vi "Find_Full_Equal_Points_and_Correct-2.vi"(4 "error IN":errorcluster, 7 "[IN] Clusters for Re\nconstructed Tracks":T1) -> (0 "error OUT":errorcluster, 3 "[OUT] Clusters for Re\nconstructed Tracks":T1)   [LabVIEW 2013]
doc: "The subVI corrects observed problem with reconstructing of resolved tracks: time-to-time, in severe conditions (big max displacement, many objects), the problem with copying of resolved subtracks"
panel:
  out "# of Track":i32
  out "Index in Track":i32
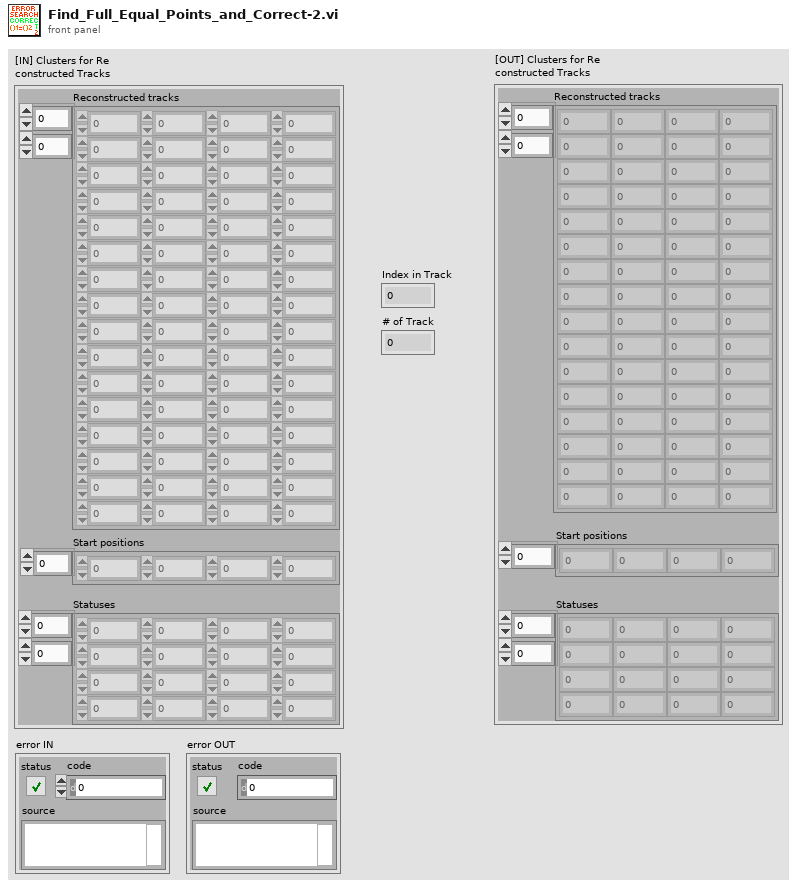
[diagram p1: front panel]
types:
  T1 = cluster{"Reconstructed tracks":dbl[][], "Start positions":i32[], "Statuses":i16[][]}
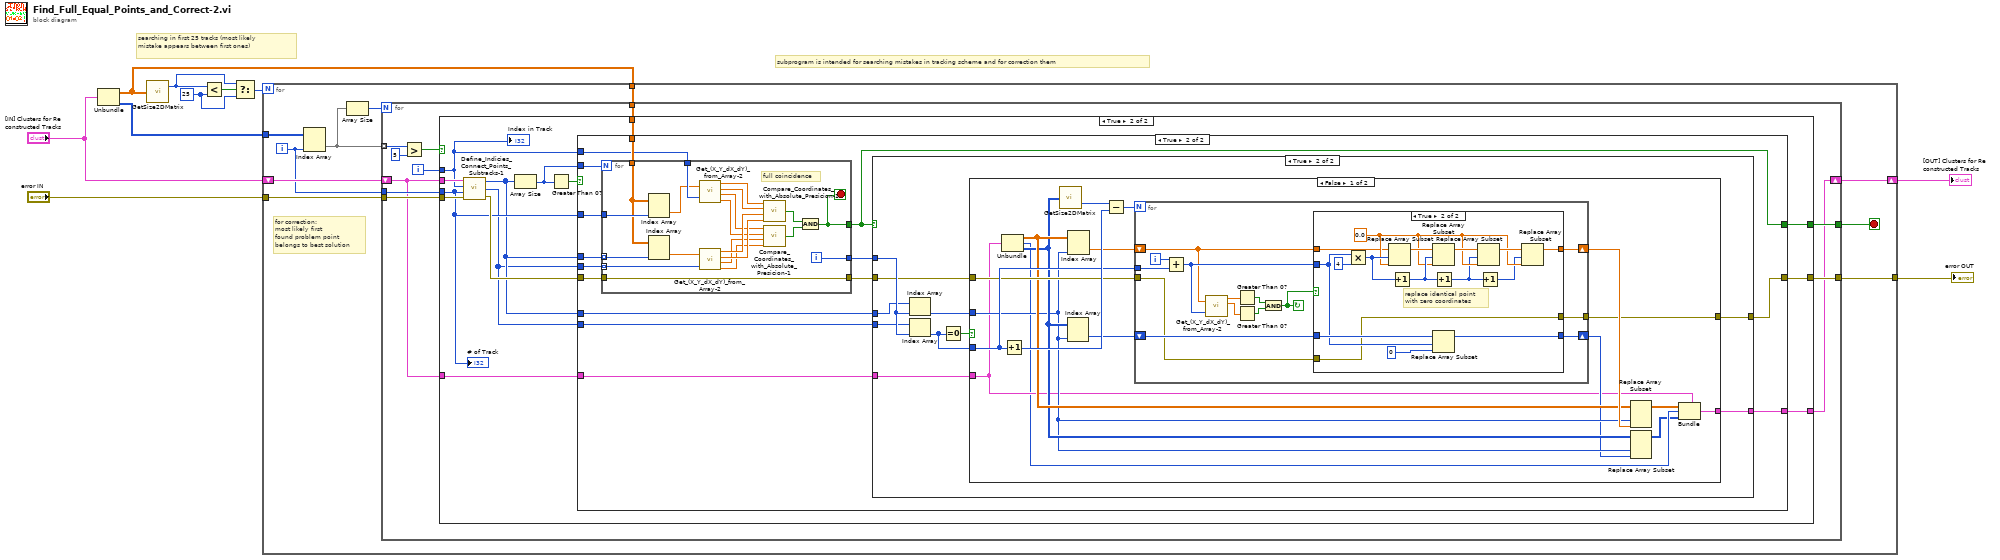
[diagram p0: block diagram]
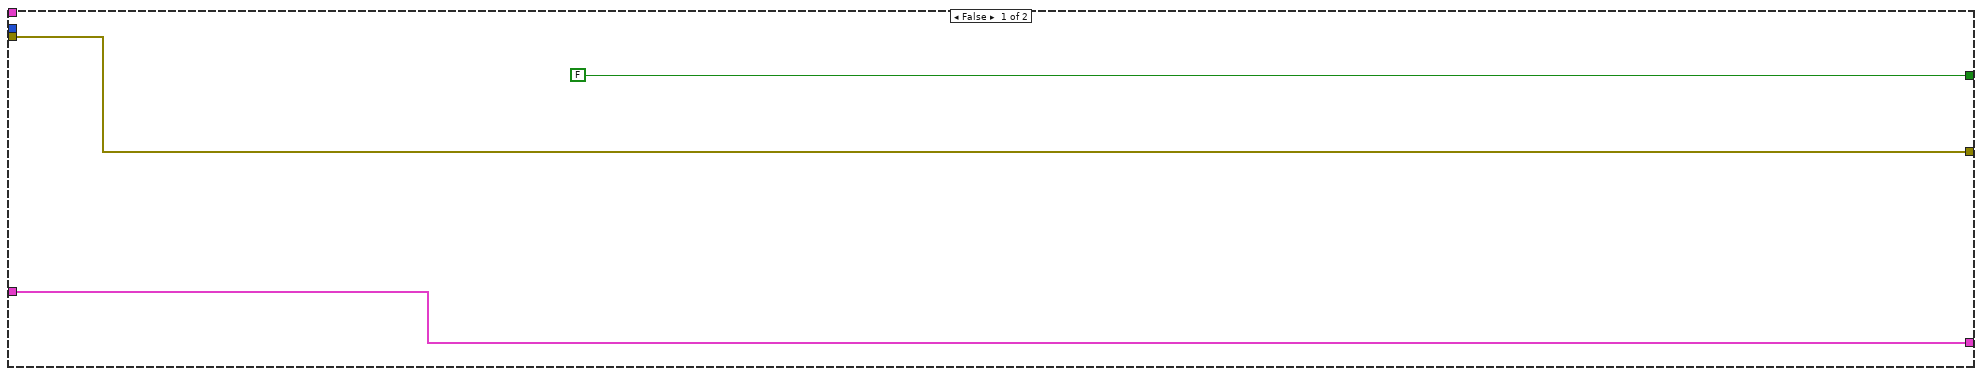
[diagram p2: hidden frame]
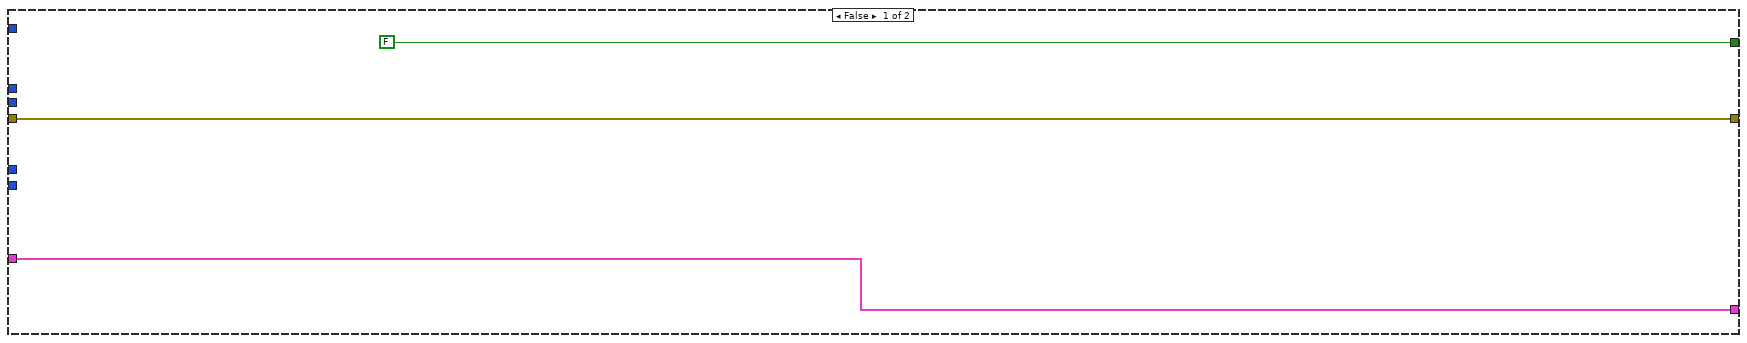
[diagram p3: hidden frame]
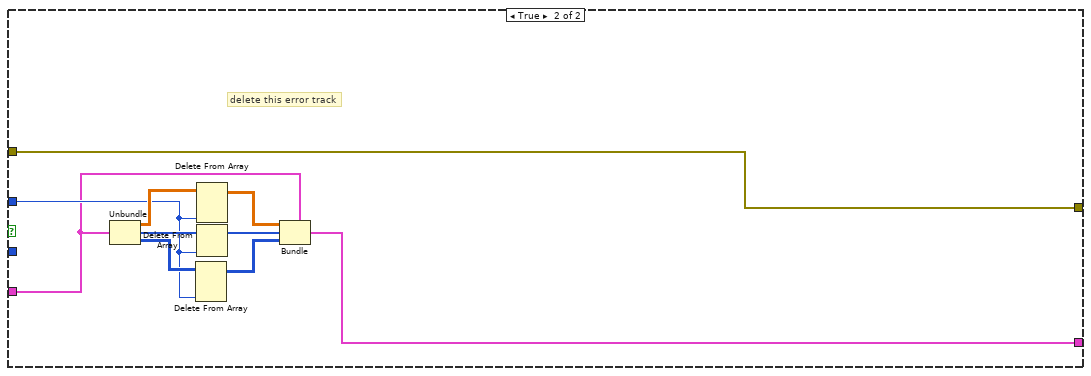
[diagram p6: hidden frame]
diagram:
  w4 = 25 ("y")
  # "searching in first 25 tracks (most likely \nmistake appears between first ones)"
  # "subprogram is intended for searching mistakes in tracking scheme and for correction them"
  n1 = Unbundle("[IN] Clusters for Re\nconstructed Tracks") -> ("Reconstructed tracks"=w1:dbl[][], "Statuses"=w2:i16[][])  [unwired: 1 out]
  n2 = call "GetSize2DMatrix.vi"("Array IN (2D)"=w1) -> ("# Cols"=w5:i32)  [unwired: 1 out]
  n3 = Less?(x=w5, y=w4) -> (x < y?=w6:bool)
  n4 = Select(t=w5, s=w6, f=w4) -> (s? t:f=w3:i32)
  n5 = for {
    N: w3 -> [_]
    tunnel: w2 -> [w20]
    tunnel: "error IN" -> [w16]
    tunnel: w1 -> [w14]
    tunnel: [w12] -> w8
    shift-right: [w11] -> w7
    shift-left: "[IN] Clusters for Re\nconstructed Tracks" -> [w17]
    i -> [w15]
    stop <- w13 stop-if-true
    # "for correction:\nmost likely first\nfound problem point\nbelongs to best solution"
    n6 = Index Array(array=w20, index (col)=w15) -> (element=w18:i16[])  [unwired: 1 in]
    n7 = Array Size(array=w18) -> (size(s)=w19:i32)
    n8 = for {
      N: w19 -> [_]
      tunnel: w18 -> [w28] mode=indexing
      tunnel: w16 -> [w29]
      tunnel: w15 -> [w26]
      tunnel: w14 -> [w25]
      tunnel: [w24] -> w13
      tunnel: [w23] -> w12
      shift-right: [w21] -> w11
      shift-left: w17 -> [w22]
      i -> [w27]
      n9 = Greater?(x=w28, y=i16 5) -> (0:w30:bool)
      n10 = case shown="True" w30 {
        tunnel: w22 -> [_ w48]
        tunnel: w29 -> [w33 w47]
        tunnel: w27 -> [_ w41]
        tunnel: w26 -> [_ w42]
        tunnel: w25 -> [_ w43]
        tunnel: [FALSE w40] -> w24
        tunnel: [w33 w39] -> w23
        tunnel: w22 -> [w32 w38]
        tunnel: [w32 w35] -> w21
        frame False {
        }
        frame True {
          n11 = call "Define_Indicies_Connect_Points_Subtracks-1.vi"("error IN"=w47, "[IN] Index of track with\n(problem displacement)"=w42, "[IN] Index of problem\ndisplacement inside track"=w41, "[IN] Track group"=w48) -> ("error OUT"=w44:errorcluster, "[OUT] Index of \nconnected dots\ninside the track"=w36:i32[], "[OUT] Index of connected\ntracks with problem dot"=w37:i32[])
          n12 = Array Size(array=w37) -> (size(s)=w46:i32)
          n13 = Greater Than 0?(x=w46) -> (x > 0?=w45:bool)
          n14 = case shown="True" w45 {
            tunnel: w46 -> [_ w66]
            tunnel: w37 -> [_ w65]
            tunnel: w36 -> [_ w64]
            tunnel: w44 -> [w50 w63]
            tunnel: w43 -> [_ w62]
            tunnel: w42 -> [_ w61]
            tunnel: w41 -> [_ w60]
            tunnel: [FALSE w54] -> w40
            tunnel: [w50 w53] -> w39
            tunnel: w38 -> [w49 w59]
            tunnel: w37 -> [_ w56]
            tunnel: w36 -> [_ w55]
            tunnel: [w49 w52] -> w35
            frame False {
            }
            frame True {
              n15 = for {
                N: w66 -> [_]
                tunnel: w65 -> [w155] mode=indexing
                tunnel: w64 -> [w153] mode=indexing
                tunnel: w63 -> [w142]
                tunnel: w62 -> [w156]
                tunnel: w61 -> [w159]
                tunnel: w60 -> [w158]
                tunnel: [w141] -> w54
                tunnel: [w142] -> w57
                tunnel: [w140] -> w58
                i -> [w140]
                stop <- w141 stop-if-true
                # "full coincidence"
                n16 = Index Array(array=w156, index (col)=w159) -> (element=w157:dbl[])  [unwired: 1 in]
                n17 = Index Array(array=w156, index (col)=w155) -> (element=w154:dbl[])  [unwired: 1 in]
                n18 = call "Get_(X_Y_dX_dY)_from_Array-2.vi"("(X,Y,dX,dY)"=w157, "Index of Displacement"=w158) -> ("X"=w152:dbl, "Y"=w151:dbl, "dX"=w148:dbl, "dY"=w147:dbl)
                n19 = call "Get_(X_Y_dX_dY)_from_Array-2.vi"("(X,Y,dX,dY)"=w154, "Index of Displacement"=w153) -> ("X"=w150:dbl, "Y"=w149:dbl, "dX"=w146:dbl, "dY"=w145:dbl)
                n20 = call "Compare_Coordinates_with_Absolute_Presicion-1.vi"("X 1"=w152, "Y 1"=w151, "X 2"=w150, "Y 2"=w149) -> ("[OUT] Same coordinates?"=w144:bool)  [unwired: 1 in]
                n21 = call "Compare_Coordinates_with_Absolute_Presicion-1.vi"("X 1"=w148, "Y 1"=w147, "X 2"=w146, "Y 2"=w145) -> ("[OUT] Same coordinates?"=w143:bool)  [unwired: 1 in]
                n22 = And(x=w144, y=w143) -> (x .and. y?=w141:bool)
              }
              n23 = case shown="True" w54 {
                tunnel: w59 -> [w68 w78]
                tunnel: w58 -> [_ w77]
                tunnel: w57 -> [w67 w76]
                tunnel: w56 -> [_ w75]
                tunnel: w55 -> [_ w74]
                tunnel: [w68 w70] -> w52
                tunnel: [w67 w69] -> w53
                frame False {
                }
                frame True {
                  n24 = Index Array(array=w75, index=w77) -> (element=w72:i32)
                  n25 = Index Array(array=w74, index=w77) -> (element=w71:i32)
                  n26 = Equal To 0?(x=w71) -> (x = 0?=w73:bool)
                  n27 = case shown="False" w73 {
                    tunnel: w76 -> [w90 w130]
                    tunnel: w78 -> [w84 w135]
                    tunnel: w72 -> [w86 w136]
                    tunnel: [w80 w131] -> w70
                    tunnel: w71 -> [w92 _]
                    tunnel: [w79 w130] -> w69
                    frame False {
                      n28 = Unbundle(w84) -> ("Reconstructed tracks"=w88:dbl[][], "Start positions"=w82:i32[], "Statuses"=w87:i16[][])
                      n29 = Increment(x=w92) -> (x+1=w95:i32)
                      n30 = call "GetSize2DMatrix.vi"("Array IN (2D)"=w87) -> ("# Rows"=w96:i32)  [unwired: 1 out]
                      n31 = Index Array(array=w87, index (col)=w86) -> (element=w91:i16[])  [unwired: 1 in]
                      n32 = Index Array(array=w88, index (col)=w86) -> (element=w93:dbl[])  [unwired: 1 in]
                      n33 = Subtract(x=w96, y=w95) -> (x-y=w94:i32)
                      n34 = for {
                        N: w94 -> [_]
                        shift-right: [w108] -> w89
                        shift-left: w93 -> [w104]
                        tunnel: w92 -> [w109]
                        shift-right: [w99] -> w85
                        shift-left: w91 -> [w100]
                        tunnel: w90 -> [w98]
                        tunnel: [w97] -> w79
                        i -> [w110]
                        stop <- w101 continue-if-true
                        n35 = Add(x=w110, y=w109) -> (x+y=w107:i32)
                        n36 = call "Get_(X_Y_dX_dY)_from_Array-2.vi"("(X,Y,dX,dY)"=w104, "Index of Displacement"=w107) -> ("X"=w106:dbl, "Y"=w105:dbl)  [unwired: 2 out]
                        n37 = Greater Than 0?(x=w106) -> (x > 0?=w103:bool)
                        n38 = Greater Than 0?(x=w105) -> (x > 0?=w102:bool)
                        n39 = And(x=w103, y=w102) -> (x .and. y?=w101:bool)
                        n40 = case shown="True" w101 {
                          tunnel: [w113 w120] -> w108
                          tunnel: w107 -> [_ w117]
                          tunnel: w104 -> [w113 w119]
                          tunnel: w100 -> [w112 w118]
                          tunnel: [w112 w115] -> w99
                          tunnel: w98 -> [w111 w114]
                          tunnel: [w111 w114] -> w97
                          frame False {
                          }
                          frame True {
                            w123 = 0.0 ("new element/subarray")
                            # "replace identical point \nwith zero coordinates"
                            n41 = Multiply(x=w117, y=4) -> (x*y=w127:i32)
                            n42 = Replace Array Subset(array=w119, new element=w123, index=w127) -> (w128:dbl[])
                            n43 = Increment(x=w127) -> (x+1=w125:i32)
                            n44 = Replace Array Subset(array=w128, new element=w123, index=w125) -> (w126:dbl[])
                            n45 = Replace Array Subset(array=w118, new element=i16 0 ("new element/subarray"), index=w117) -> (w115:i16[])
                            n46 = Increment(x=w125) -> (x+1=w122:i32)
                            n47 = Replace Array Subset(array=w126, new element=w123, index=w122) -> (w124:dbl[])
                            n48 = Increment(x=w122) -> (x+1=w121:i32)
                            n49 = Replace Array Subset(array=w124, new element=w123, index=w121) -> (w120:dbl[])
                          }
                        }
                      }
                      n50 = Replace Array Subset(array=w88, new element=w89, index (col)=w86) -> (w83:dbl[][])  [unwired: 1 in]
                      n51 = Replace Array Subset(array=w87, new element=w85, index (col)=w86) -> (w81:i16[][])  [unwired: 1 in]
                      n52 = Bundle(cluster=w84, "Reconstructed tracks"=w83, "Start positions"=w82, "Statuses"=w81) -> (w80:T1)
                    }
                    frame True {
                      # "delete this error track"
                      n53 = Unbundle(w135) -> ("Reconstructed tracks"=w139:dbl[][], "Start positions"=w138:i32[], "Statuses"=w137:i16[][])
                      n54 = Delete From Array(array=w137, index (col)=w136) -> (array with subset deleted=w132:i16[][])  [unwired: 2 in, 1 out]
                      n55 = Delete From Array(array=w139, index (col)=w136) -> (array with subset deleted=w134:dbl[][])  [unwired: 2 in, 1 out]
                      n56 = Delete From Array(array=w138, index=w136) -> (array with subset deleted=w133:i32[])  [unwired: 1 in, 1 out]
                      n57 = Bundle(cluster=w135, "Reconstructed tracks"=w134, "Start positions"=w133, "Statuses"=w132) -> (w131:T1)
                    }
                  }
                }
              }
            }
          }
          "Index in Track" <- w41
          "# of Track" <- w42
        }
      }
    }
  }
  "error OUT" <- w8
  "[OUT] Clusters for Re\nconstructed Tracks" <- w7
